vi "RT Host.vi"() -> ()   [LabVIEW 2017]
uses:
  <vilib>/Instr/_visa.llb/VISA Configure Serial Port (Instr).vi
panel:
  out "XY Graph":cluster{dbl[], dbl[]}(graph)
  out "error out":errorcluster
  in  "milliseconds to wait":u32=50
  out "Enc 0 angle (rad)":dbl
  out "Enc 1 angle (rad)":dbl
  out "Encoder1":i32
  out "Encoder0":i32
  out "Link2Y":dbl
  out "Link2X":dbl
  out "Link1Y":dbl
  out "Link1X":dbl
  in  "stop":bool
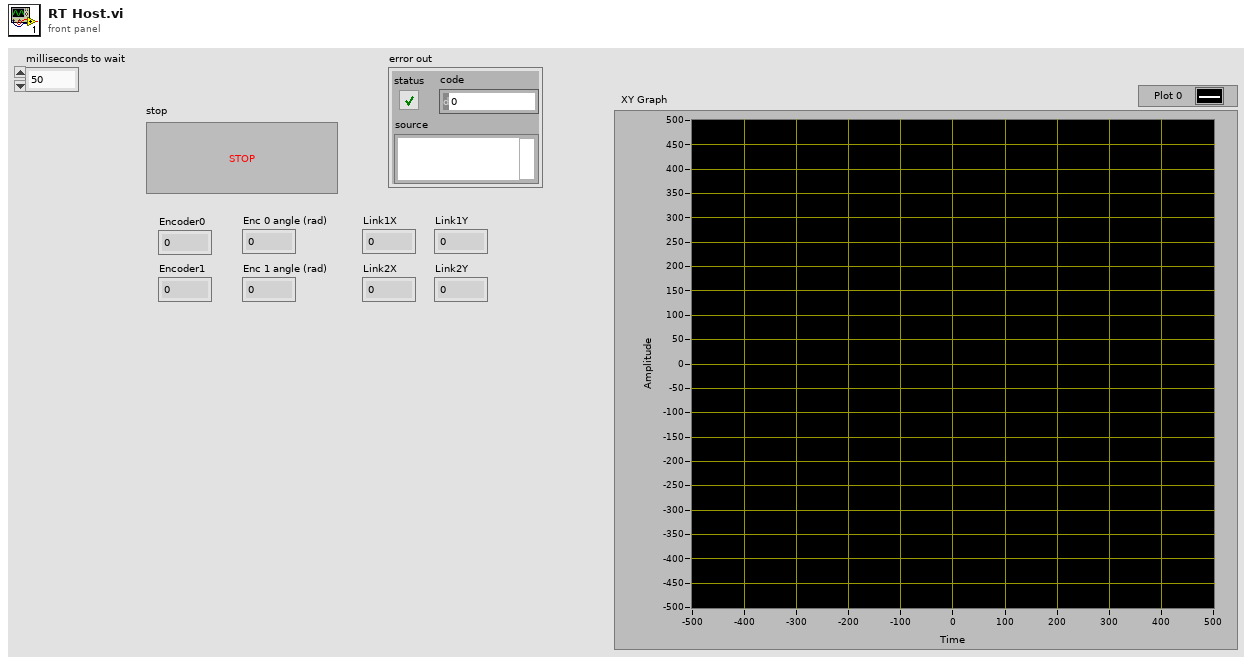
[diagram p1: front panel]
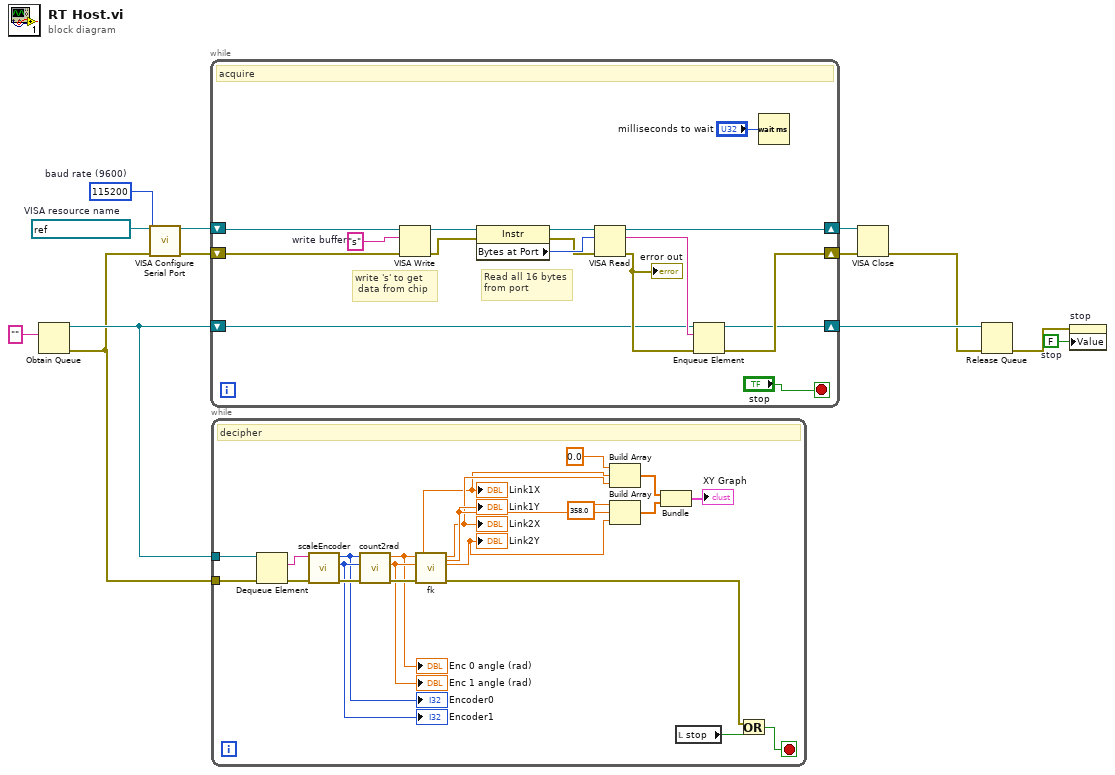
[diagram p0: block diagram]
diagram:
  w1 = FALSE  # stop
  w12 = u32 115200  # baud rate (9600)
  w13 = refnum<visa-resource-name> "ASRL2::INSTR"  # VISA resource name
  n1 = Obtain Queue(element data type="") -> (queue out=w8:refnum<queue>, error out=w7:errorcluster)  [unwired: 4 in, 1 out]
  n2 = call-poly "VISA Configure Serial Port"("VISA resource name"=w13, "baud rate (9600)"=w12, "error in (no error)"=w7) -> ("VISA resource name out"=w11:refnum<visa-resource-name>, "error out"=w10:errorcluster)  [unwired: 11 in]
  n3 = while {
    shift-right: [w19] -> w5
    shift-left: w11 -> [w22]
    shift-right: [w18] -> w6
    shift-left: w10 -> [w23]
    shift-right: [w16] -> w4
    shift-left: w8 -> [w17]
    stop <- "stop" stop-if-true
    w29 = "s"  # write buffer
    # "Read all 16 bytes\nfrom port"
    # "write 's' to get\n data from chip"
    # "acquire"
    n4 = VISA Write(VISA resource name=w22, write buffer=w29, error in (no error)=w23) -> (VISA resource name out=w28:refnum<visa-resource-name>, error out=w27:errorcluster)  [unwired: 1 out]
    n5 = property class="Instr"(reference=w28, error in=w27) -> (reference out=w25:refnum<visa-resource-name>, error out=w24:errorcluster, "Bytes at Port"=w26:u32)
    n6 = VISA Read(VISA resource name=w25, byte count=w26, error in (no error)=w24) -> (VISA resource name out=w19:refnum<visa-resource-name>, read buffer=w20:string, error out=w21:errorcluster)  [unwired: 1 out]
    "error out" <- w21
    n7 = Enqueue Element(queue=w17, element=w20, error in (no error)=w21) -> (queue out=w16:refnum<queue>, error out=w18:errorcluster)  [unwired: 1 in, 1 out]
    n8 = Wait (ms)(milliseconds to wait="milliseconds to wait") -> ()  [unwired: 1 out]
  }
  n9 = while {
    tunnel: w8 -> [w51]
    tunnel: w7 -> [w50]
    stop <- w49 stop-if-true
    # "decipher"
    n10 = Dequeue Element(queue=w51, error in (no error)=w50) -> (element=w48:string, error out=w47:errorcluster)  [unwired: 1 in, 2 out]
    n11 = call "scaleEncoder.vi"("error in (no error)"=w47, "String"=w48) -> ("error out"=w46:errorcluster, "Encoder1"=w45:i32, "Encoder0"=w44:i32)  [unwired: 7 in]
    "Encoder0" <- w44
    "Encoder1" <- w45
    n12 = call "count2rad.vi"("error in (no error)"=w46, "Encoder 1 Count"=w45, "Encoder 0 Count"=w44) -> ("error out"=w43:errorcluster, "Enc 1 angle (rad)"=w42:dbl, "Enc 0 angle (rad)"=w41:dbl)  [unwired: 6 in]
    "Enc 1 angle (rad)" <- w42
    "Enc 0 angle (rad)" <- w41
    n13 = call "fk.vi"("error in (no error)"=w43, "Theta 1"=w42, "Theta 0"=w41) -> ("error out"=w40:errorcluster, "Link2Y"=w37:dbl, "Link2X"=w36:dbl, "Link1Y"=w38:dbl, "Link1X"=w35:dbl)  [unwired: 4 in]
    "Link1X" <- w35
    "Link1Y" <- w38
    "Link2X" <- w36
    "Link2Y" <- w37
    n14 = Build Array(0.0, w35, w36) -> (w32:dbl[])
    n15 = Build Array(358.0, w38, w37) -> (w31:dbl[])
    n16 = Bundle(w32, w31) -> (→"XY Graph":cluster{dbl[], dbl[]})  [unwired: 1 in]
    n17 = local read "stop"() -> (w39:bool)
    n18 = Or(x=w40, y=w39) -> (x .or. y?=w49:bool)
  }
  n19 = VISA Close(VISA resource name=w5, error in (no error)=w6) -> (error out=w3:errorcluster)
  n20 = Release Queue(queue=w4, error in (no error)=w3) -> (error out=w2:errorcluster)  [unwired: 1 in, 2 out]
  n21 = property on="stop" class="Bool (strict)"(error in=w2, "Value"=w1) -> ()  [unwired: 1 in, 2 out]
